vi "AddParametersToSweepResults.vi"(8 "error in (no error)":errorcluster, 9 "SweepResults [i]":T1, 10 "AO":waveform(dbl)[](array[waveform]), 11 "LockinDAQ in":refnum<class "Lockin.DAQ.lvclass">=refnum) -> (0 "error out":errorcluster, 1 "SweepResults [i] out":T1, 3 "LockinDAQ out":refnum<class "Lockin.DAQ.lvclass">)   [LabVIEW 2016, in "Lockin.DAQ.lvclass"]
uses:
  Lockin.DAQ.lvclass
  Typedefs/SweepResults--Cluster.ctl
  Lockin.DAQ.lvclass/Lockin.DAQ.ctl
  <vilib>/measure/NI_MAPro.lvlib
  <vilib>/measure/maresamp.llb/Resample Waveform (single shot).vi
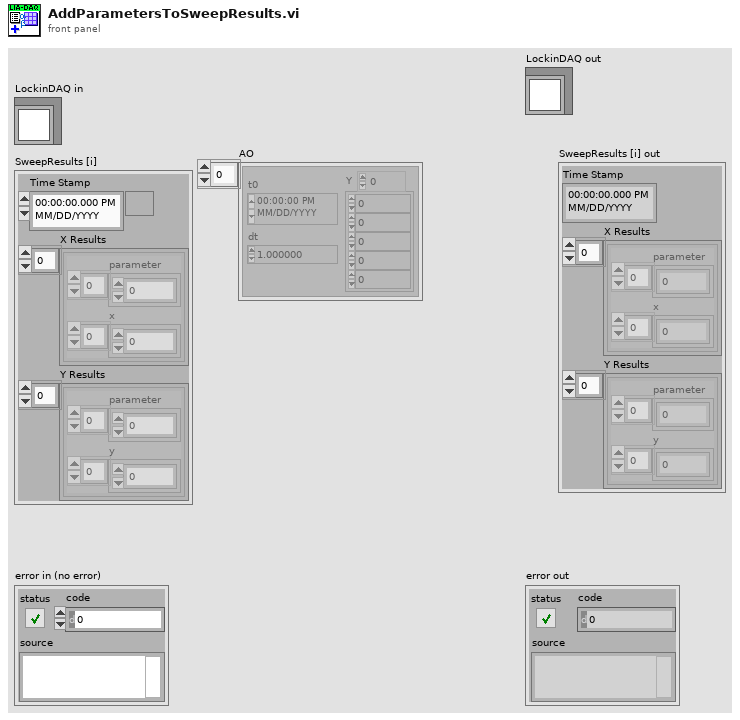
[diagram p1: front panel]
types:
  T1 = typedef "Lockin.DAQ.lvclass/SweepResults--Cluster.ctl" = cluster{"Time Stamp":timestamp, "X Results":cluster{"parameter":dbl[], "x":dbl[]}[], "Y Results":cluster{"parameter":dbl[], "y":dbl[]}[]}
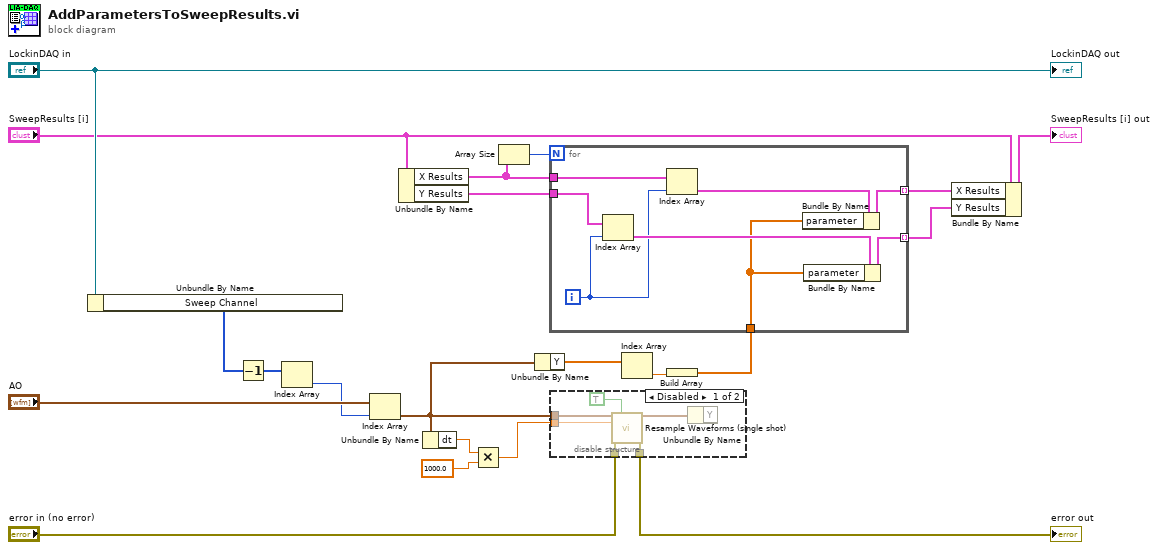
[diagram p0: block diagram]
diagram:
  n1 = Unbundle By Name("LockinDAQ in") -> ("Sweep Channel"=w16:i32[])
  n2 = Decrement(x=w16) -> (x-1=w9:i32[])
  n3 = Index Array(array=w9) -> (element=w8:i32)  [unwired: 1 in]
  n4 = Index Array(array="AO", index=w8) -> (element=w4:waveform(dbl))
  n5 = Unbundle By Name("SweepResults [i]") -> ("X Results"=w20:cluster{"parameter":dbl[], "x":dbl[]}[], "Y Results"=w21:cluster{"parameter":dbl[], "y":dbl[]}[])
  n6 = Unbundle By Name(w4) -> ("dt"=w6:dbl)
  n7 = Multiply(x=w6, y=1000.0) -> (x*y=w5:dbl)
  n8 = Array Size(array=w20) -> (size(s)=w19:i32)
  n9 = Unbundle By Name(w4) -> ("Y"=w3:dbl[])
  n10 = disable-structure shown="Disabled" {
    disable-tunnel: "error in (no error)" -> [w26 w28]
    disable-tunnel: [w25 w28] -> w10
    disable-tunnel: w5 -> [w23 _]
    disable-tunnel: w4 -> [w22 _]
    frame Disabled {
      n11 = call-poly <vilib>:"Resample Waveforms (single shot).vi"("waveform in"=w22, "open interval? (F)"=TRUE, "dt"=w23, "error in (no error)"=w26) -> ("resampled waveform out"=w27:waveform(dbl), "error out"=w25:errorcluster)  [unwired: 8 in, 2 out]
      n12 = Unbundle By Name(w27) -> ()  [unwired: 1 out]
    }
    frame Enabled {
    }
  }
  "error out" <- w10
  n13 = Index Array(array=w3) -> (element=w2:dbl)  [unwired: 1 in]
  n14 = Build Array(w2) -> (w1:dbl[])
  n15 = for {
    N: w19 -> [_]
    tunnel: [w36] -> w18 mode=indexing
    tunnel: w20 -> [w35]
    tunnel: w21 -> [w34]
    tunnel: [w33] -> w17 mode=indexing
    tunnel: w1 -> [w30]
    i -> [w29]
    n16 = Index Array(array=w34, index=w29) -> (element=w32:cluster{"parameter":dbl[], "y":dbl[]})
    n17 = Index Array(array=w35, index=w29) -> (element=w31:cluster{"parameter":dbl[], "x":dbl[]})
    n18 = Bundle By Name(cluster=w31, "parameter"=w30) -> (w36:cluster{"parameter":dbl[], "x":dbl[]})
    n19 = Bundle By Name(cluster=w32, "parameter"=w30) -> (w33:cluster{"parameter":dbl[], "y":dbl[]})
  }
  n20 = Bundle By Name(cluster="SweepResults [i]", "X Results"=w18, "Y Results"=w17) -> (→"SweepResults [i] out":T1)
  "LockinDAQ out" <- "LockinDAQ in"
